vi "Convex Hull.vi"(7 "Sort CW in 2D":bool, 8 "error in (no error)":errorcluster, 11 "points":dbl[][](array[numeric])) -> (0 "error out":errorcluster, 1 "area":dbl, 2 "volume":dbl, 3 "Simplex Indices":i32[](array[numeric]))   [LabVIEW 2019, in "QHull.lvlib"]
uses:
  QHull.lvlib
  LV_QHull_32.dll
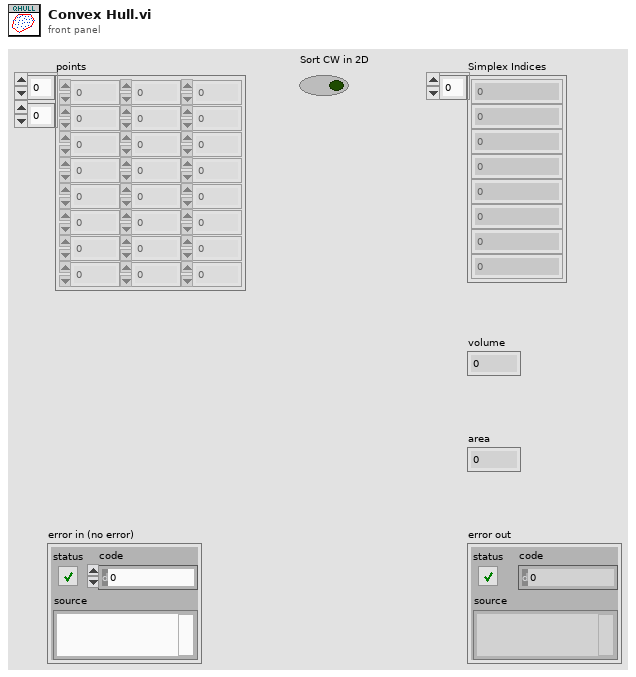
[diagram p1: front panel]
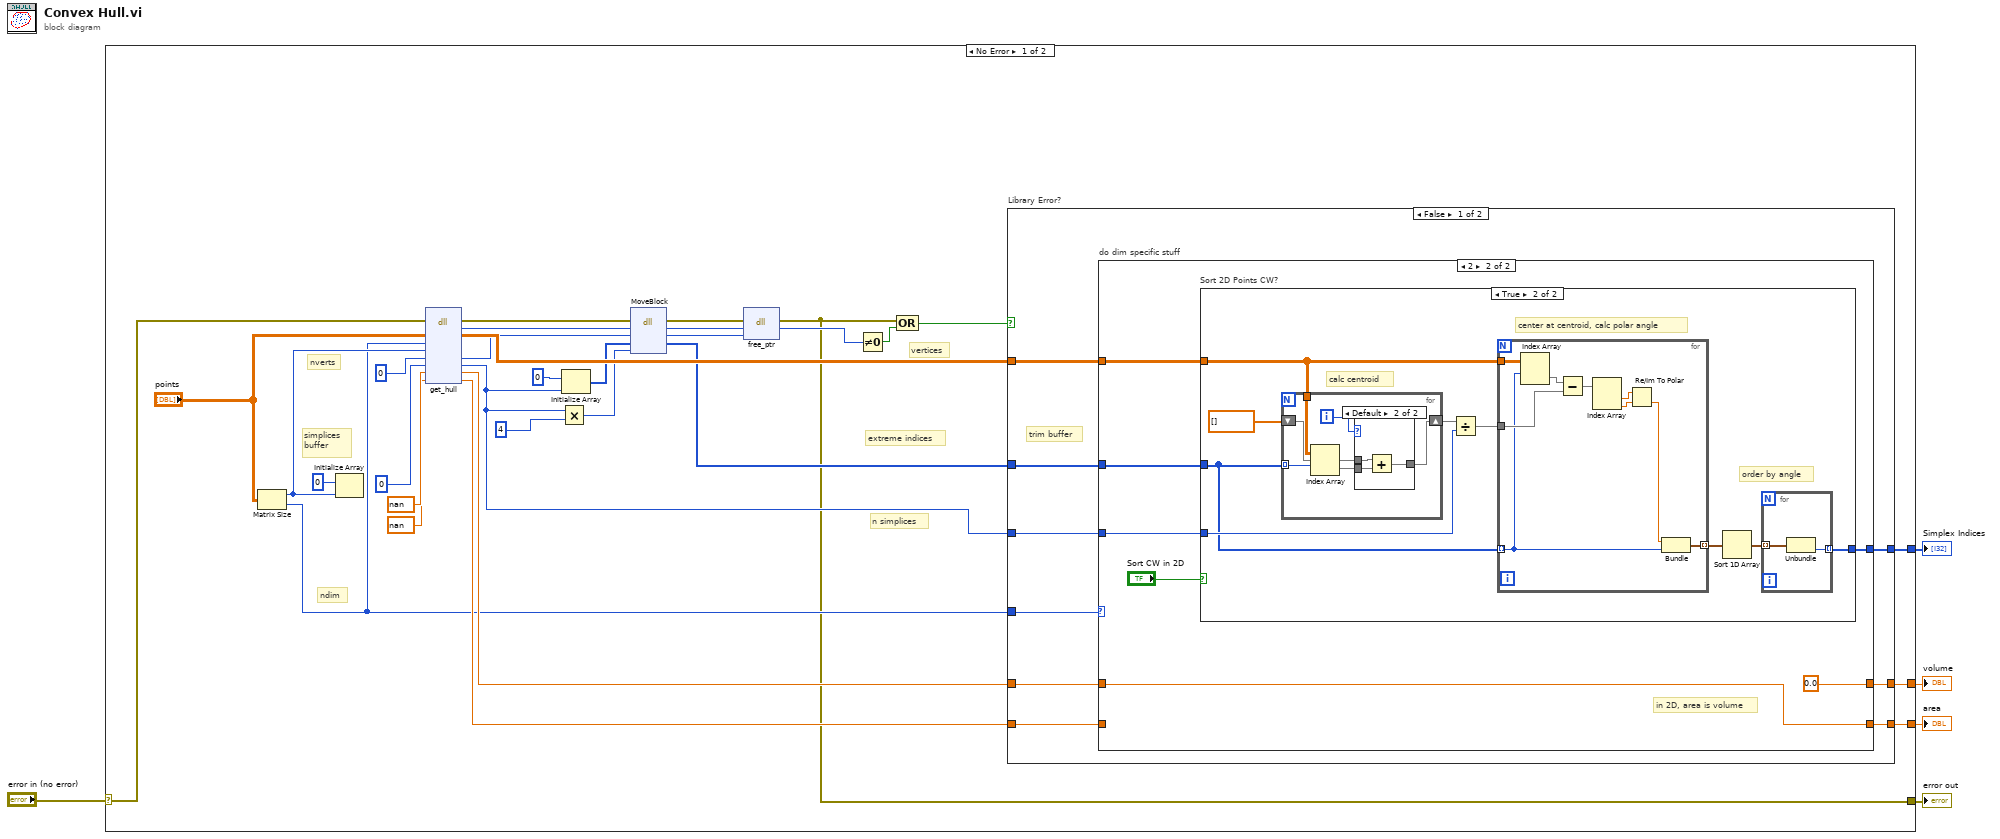
[diagram p0: block diagram]
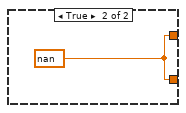
[diagram p5: hidden frame]
diagram:
  n1 = case shown="No Error" "error in (no error)" {
    selector: "error in (no error)" -> [w34 w86]
    tunnel: [w28 _] -> w4
    tunnel: [w8 w86] -> w3
    tunnel: [w22 _] -> w2
    tunnel: [w20 _] -> w1
    frame No Error {
      # "n simplices"
      # "extreme indices"
      # "vertices"
      # "simplices\nbuffer"
      # "nverts"
      # "ndim"
      n2 = Matrix Size(0:"points") -> (1:w32:i32, 2:w13:i32)
      n3 = Initialize Array(0, w32) -> ()  [unwired: 1 out]
      n4 = dll-call lib="E:/Labview/LV 2023/PPL/PPL Builder/Libs/SK Spatial/QHull/LV 2015/LV QHull/LV_QHull_*.*" fn="get_hull"(error in=w34, "points"="points", "dim"=w13, "numpoints"=w32, "simplices_ptr"=i64 0, "numsimplices"=0, "volume"=nan, "area"=nan) -> (error out=w10:errorcluster, "errorcode"=w26:i32, "points"=w27:dbl[][], "simplices_ptr"=w6:i64, "numsimplices"=w14:i32, "volume"=w23:dbl, "area"=w21:dbl)  [unwired: 4 in, 1 out]
      n5 = Multiply(x=w14, y=4 ("value")) -> (x*y=w15:i32)
      n6 = Initialize Array(0 ("element"), w14) -> (w16:i32[])
      n7 = dll-call lib="LabVIEW" fn="MoveBlock"(error in=w10, "ps"=w6, "pd"=w16, "size"=w15) -> (error out=w9:errorcluster, "ps"=w7:i64, "pd"=w11:i32[])  [unwired: 4 in, 1 out]
      n8 = dll-call lib="E:/Labview/LV 2023/PPL/PPL Builder/Libs/SK Spatial/QHull/LV 2015/LV QHull/LV_QHull_*.*" fn="free_ptr"(error in=w9, "ptr"=w7) -> (error out=w8:errorcluster)  [unwired: 4 in, 1 out]
      n9 = Not Equal To 0?(x=w26) -> (x != 0?=w25:bool)
      n10 = Compound Arithmetic op=OR(w8, w25) -> (w24:bool)
      n11 = case "Library Error?" shown="False" w24 {
        tunnel: w14 -> [w43 _]
        tunnel: [w42 _] -> w28
        tunnel: w13 -> [w39 _]
        tunnel: w27 -> [w41 _]
        tunnel: w23 -> [w36 _]
        tunnel: [w37 w85] -> w22
        tunnel: w21 -> [w40 _]
        tunnel: [w38 w85] -> w20
        tunnel: w11 -> [w35 _]
        frame False {
          # "trim buffer"
          n12 = case "do dim specific stuff" shown="2" w39 {
            tunnel: w43 -> [_ w53]
            tunnel: w35 -> [w46 w52]
            tunnel: [w46 w50] -> w42
            tunnel: w41 -> [_ w49]
            tunnel: w40 -> [w44 _]
            tunnel: [w44 w47] -> w38
            tunnel: [w45 0.0 ("t")] -> w37
            tunnel: w36 -> [w45 w47]
            frame Default {
            }
            frame 2 {
              # "in 2D, area is volume"
              n13 = case "Sort 2D Points CW?" shown="True" "Sort CW in 2D" {
                tunnel: w53 -> [_ w61]
                tunnel: w49 -> [_ w55]
                tunnel: w52 -> [w54 w60]
                tunnel: [w54 w56] -> w50
                frame False {
                }
                frame True {
                  # "order by angle"
                  # "center at centroid, calc polar angle"
                  # "calc centroid"
                  n14 = for {
                    tunnel: w55 -> [w80]
                    tunnel: w60 -> [w79] mode=indexing
                    shift-right: [w77] -> w62
                    shift-left: dbl[] [] ("points") -> [w76]
                    i -> [w75]
                    n15 = Index Array(array=w80, index (row)=w79) -> (element=w78:dbl[])  [unwired: 1 in]
                    n16 = case shown="Default" w75 {
                      tunnel: w78 -> [w81 w84]
                      tunnel: [w81 w83] -> w77
                      tunnel: w76 -> [_ w82]
                      frame 0 {
                      }
                      frame Default {
                        n17 = Add(x=w82, y=w84) -> (x+y=w83:dbl[])
                      }
                    }
                  }
                  n18 = Divide(x=w62, y=w61) -> (x/y=w59:dbl[])
                  n19 = for {
                    tunnel: w55 -> [w74]
                    tunnel: w60 -> [w67] mode=indexing
                    tunnel: w59 -> [w72]
                    tunnel: [w66] -> w58 mode=indexing
                    n20 = Index Array(array=w74, index (row)=w67) -> (element=w73:dbl[])  [unwired: 1 in]
                    n21 = Subtract(x=w73, y=w72) -> (x-y=w71:dbl[])
                    n22 = Index Array(array=w71) -> (element #1=w70:dbl, element #2=w69:dbl)  [unwired: 2 in]
                    n23 = Re/Im To Polar(2:w69, 3:w70) -> (0:w68:dbl)  [unwired: 1 out]
                    n24 = Bundle(w68, w67) -> (w66:cluster{dbl, i32})  [unwired: 1 in]
                  }
                  n25 = Sort 1D Array(array=w58) -> (sorted array=w57:cluster{dbl, i32}[])
                  n26 = for {
                    tunnel: w57 -> [w65] mode=indexing
                    tunnel: [w64] -> w56 mode=indexing
                    n27 = Unbundle(w65) -> (w64:i32)  [unwired: 1 out]
                  }
                }
              }
            }
          }
        }
        frame True {
          w85 = nan ("volume")
        }
      }
    }
    frame Error {
    }
  }
  "Simplex Indices" <- w4
  "error out" <- w3
  "volume" <- w2
  "area" <- w1
